vi "Get Table for Testing.vi"(8 "error in (no error)":errorcluster, 11 "Open Close Logic Simple Table in":refnum<class "Open Close Logic Simple Table.lvclass">) -> (0 "error out":errorcluster, 1 "Nested":T1[](array[typedef]), 2 "Caller":T1[](array[typedef]), 3 "Open Close Logic Simple Table out":refnum<class "Open Close Logic Simple Table.lvclass">)   [LabVIEW 2020, in "Open Close Logic Simple Table.lvlib" / "Open Close Logic Simple Table.lvclass"]
uses:
  Open Close Logic Simple Table.lvclass
  Autoclose manager/Form ID.ctl
  Open Close Logic Simple Table.lvclass/Open Close Logic Simple Table.ctl
  Form Server Interfaces.lvlib
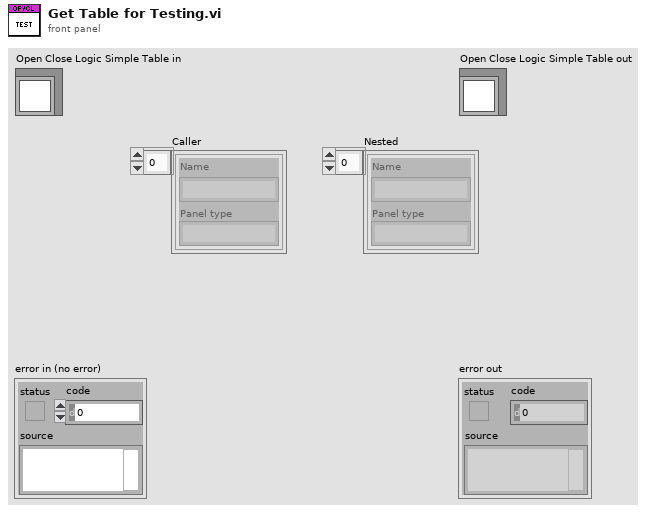
[diagram p1: front panel]
types:
  T1 = typedef "Form Server Interfaces.lvlib/Form ID.ctl" = cluster{"Name":string, "Panel type":string}
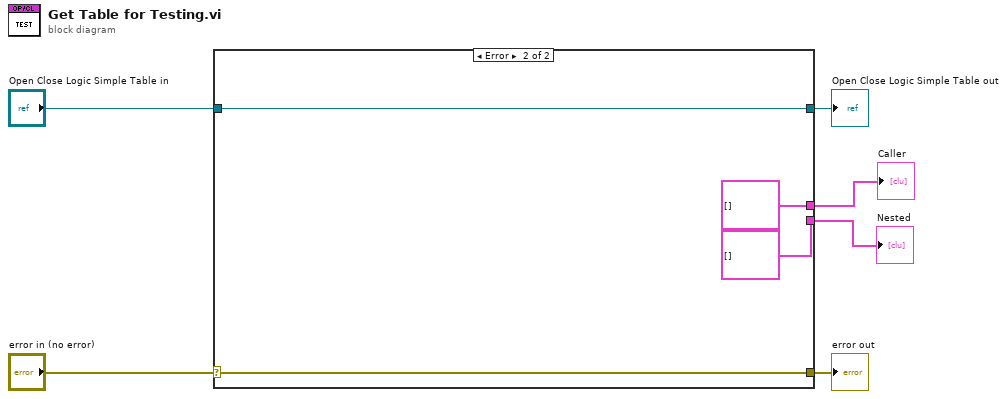
[diagram p0: block diagram]
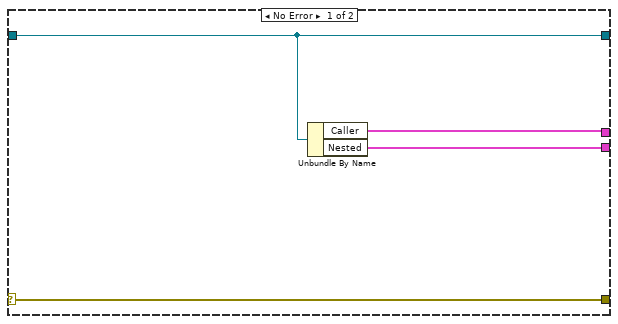
[diagram p2: hidden frame]
diagram:
  n1 = case shown="Error" "error in (no error)" {
    selector: "error in (no error)" -> [w10 w14]
    tunnel: [w10 w14] -> w5
    tunnel: [w9 w13] -> w3
    tunnel: "Open Close Logic Simple Table in" -> [w9 w13]
    tunnel: [w8 T1[] [] ("Caller")] -> w2
    tunnel: [w7 T1[] [] ("Nested")] -> w1
    frame No Error {
      n2 = Unbundle By Name(w9) -> ("Caller"=w8:T1[], "Nested"=w7:T1[])
    }
    frame Error {
    }
  }
  "error out" <- w5
  "Open Close Logic Simple Table out" <- w3
  "Caller" <- w2
  "Nested" <- w1
